vi "General Gaussian Monopulse.vi"(5 "X":dbl[](array[numeric]), 7 "center frequency":dbl=0.1, 8 "delta t":dbl=0.1, 9 "delay":dbl, 10 "amplitude":dbl=1.0, 11 "samples":i32=128) -> (0 "error":i32, 3 "Gaussian Monopulse":dbl[](array[numeric]))   [LabVIEW 2017, in "NI_AALBase.lvlib"]
uses:
  NI_AALBase.lvlib
  lvanlys.dll
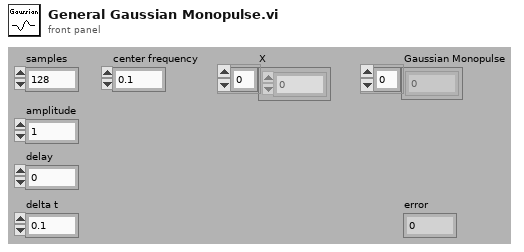
[diagram p1: front panel]
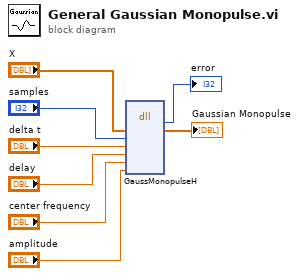
[diagram p0: block diagram]
diagram:
  n1 = dll-call lib="C:/Program Files/National Instruments/LabVIEW 2017/resource/lvanlys.*" fn="GaussMonopulseH"("x"="X", "samples"="samples", "delta"="delta t", "delay"="delay", "fc"="center frequency", "amp"="amplitude") -> ("error"=→"error":i32, "x"=→"Gaussian Monopulse":dbl[])  [unwired: 8 in, 2 out]
